vi "VISA test.vi"() -> ()   [LabVIEW 2012]
uses:
  <vilib>/Instr/_visa.llb/VISA Find Search Mode.ctl
  <vilib>/Platform/TimedLoop/XDataNode/timing_clust.ctl
  <vilib>/Platform/TimedLoop/XDataNode/nitl_modes.ctl
  <vilib>/Platform/TimedLoop/XDataNode/wakeup.ctl
  <vilib>/Instr/_visa.llb/VISA Configure Serial Port (Instr).vi
  <vilib>/Platform/TimedLoop/XDataNode/XDataNode.xnode
  <vilib>/Platform/TimedLoop/XDataNode/XDNodeRunTimeDep.lvlib
panel:
  in  "data3":string
  in  "data2":string
  out "Actual polling freq. (Hz)":dbl=10.0
  in  "stop":bool
  in  "Poll freq.(Hz)":dbl=10.0
  in  "data1":string
  in  "cmd":string="2"
  in  "add":u8=1
  out "Checksum ok?":bool=TRUE
  out "chk":u8=183 format="%x"
  out "term":string="\r"
  out "Output to device":string="$012B7\r"
  in  "bytes to read":u32=64
  in  "flow control (0:none)":u16(ring) items=["None", "XON/XOFF", "RTS/CTS", "XON/XOFF & RTS/CTS", "DTR/DSR", "XON/XOFF & DTR/DSR"]
  in  "stop bits":u16(ring)=10 items=["1.0"=10, "1.5"=15, "2.0"=20]
  in  "parity":enum16{"None", "Odd", "Even", "Mark", "Space"}(ring)
  in  "data bits":u16=8 min=5 max=8 step=1
  in  "baud rate (bps)":u32=9600
  in  "timeout (ms)":u32=1000
  in  "enable termination char":bool=TRUE
  in  "termination char":u8=13 format="%.0x"
  out "bytes returned":u32=12
  out "Error":errorcluster
  out "Response from device":string="!010806C0C3\r"
  out "bytes written":u32=7
  in  "del":string="$"
  in  "VISA resource name":refnum<visa-resource-name>="COM3"
  out "Port list":string[](array[string])=["COM1", "COM3"]
  # "(hex)"
  # "(hex)"
  # "(dec)"
  # "(hex)"
  # "(hex)"
  # "(hex)"
  # "(str)"
  # "(str)"
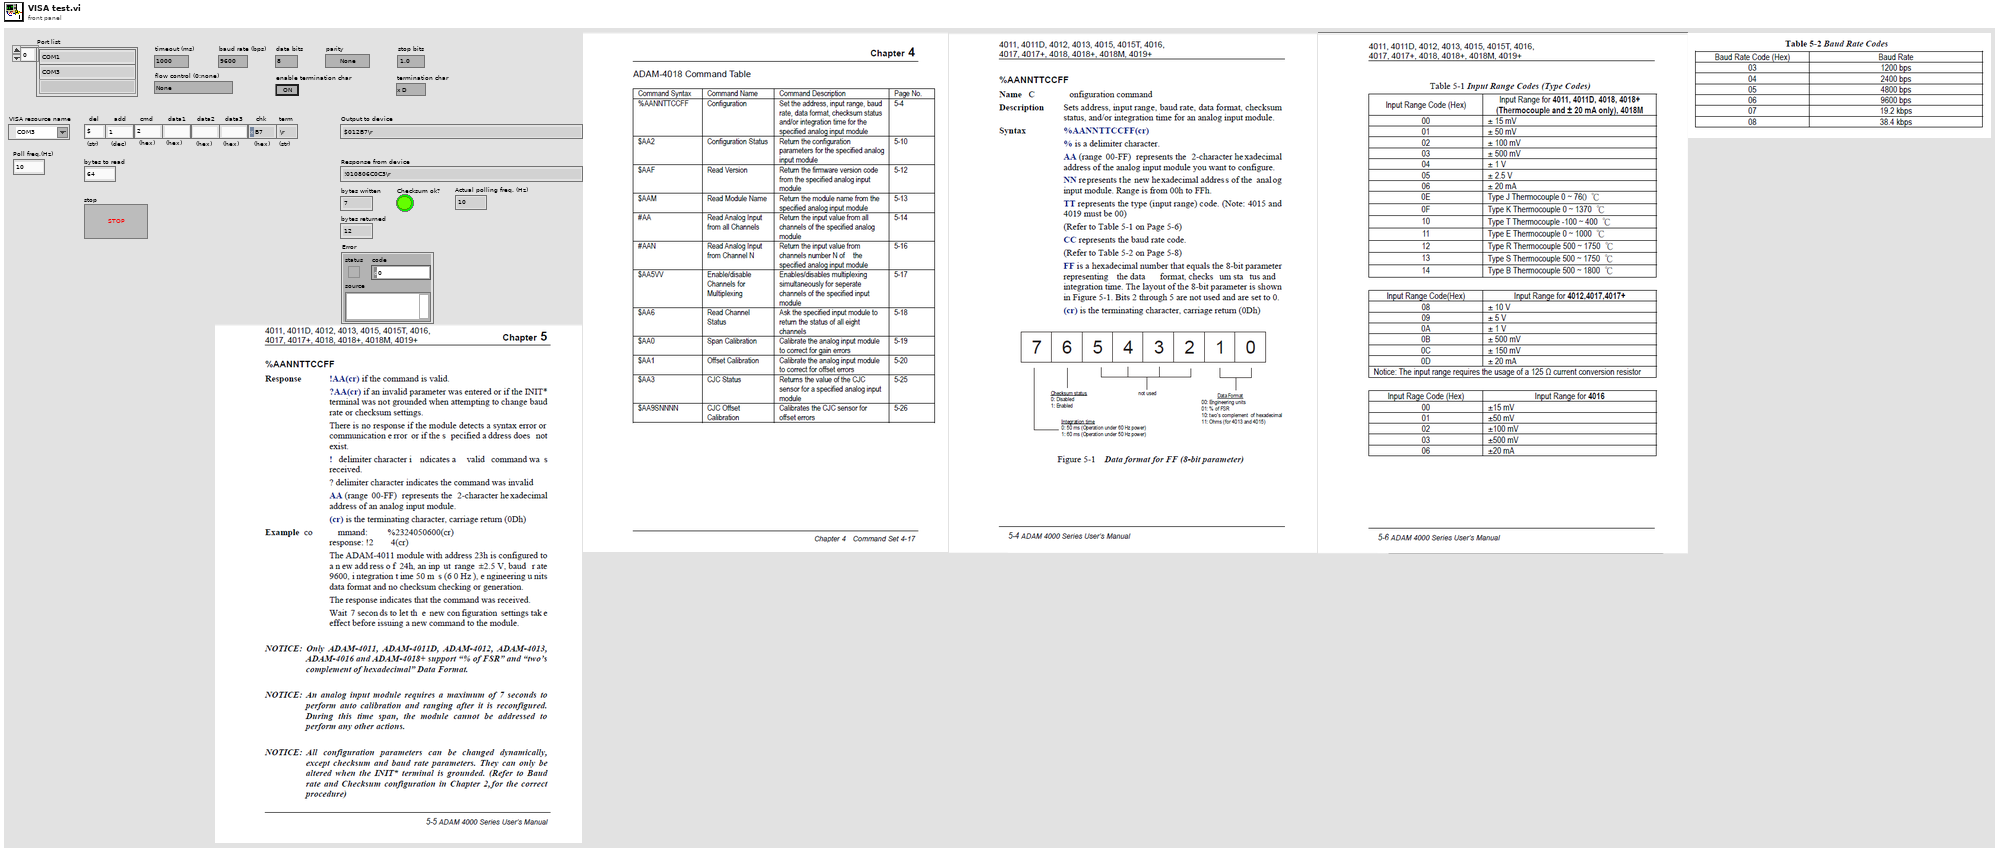
[diagram p1: front panel]
types:
  T1 = typedef "VISA Find Search Mode.ctl" = u32
  T2 = typedef "XDNodeRunTimeDep.lvlib/timing_clust.ctl" = cluster{"Expected End [f-1]":u64, "Actual End [f-1]":u64, "Finished Late? [f-1]":bool, "Expected End [i-1]":u64, "Actual End [i-1]":u64, "Finished Late? [i-1]":bool, "Expected Start [i]":u64, "Actual Start [i]":u64, "Expected Start [f]":u64, "Actual Start [f]":u64, "Source Name":string, "Structure Name":string, "Period":i64, "Deadline":i64, "Offset":i64, "Start":i64, "Priority":i32, "Timeout":i32, "Mode":T3, "Wakeup Reason":T4, "Error":errorcluster, "Source Type":string, "Secondary Source Type":string, "Global End Time":u64, "Global Start Time":u64, "Frame Duration":u64, "Iteration Duration":u64, "Assigned CPU":i32, "I/O Scan Engine Mode":u32}
  T3 = typedef "XDNodeRunTimeDep.lvlib/nitl_modes.ctl" = enum32{"No Change", "Process missed periods, maintain original phase", "Discard missed periods, maintain original phase", "Process missed periods, ignore original phase", "Discard missed periods, ignore original phase"}
  T4 = typedef "XDNodeRunTimeDep.lvlib/wakeup.ctl" = enum32{"Normal", "Aborted", "Asynchronous wakeup", "Timing source error", "Timed loop error", "Timeout"}
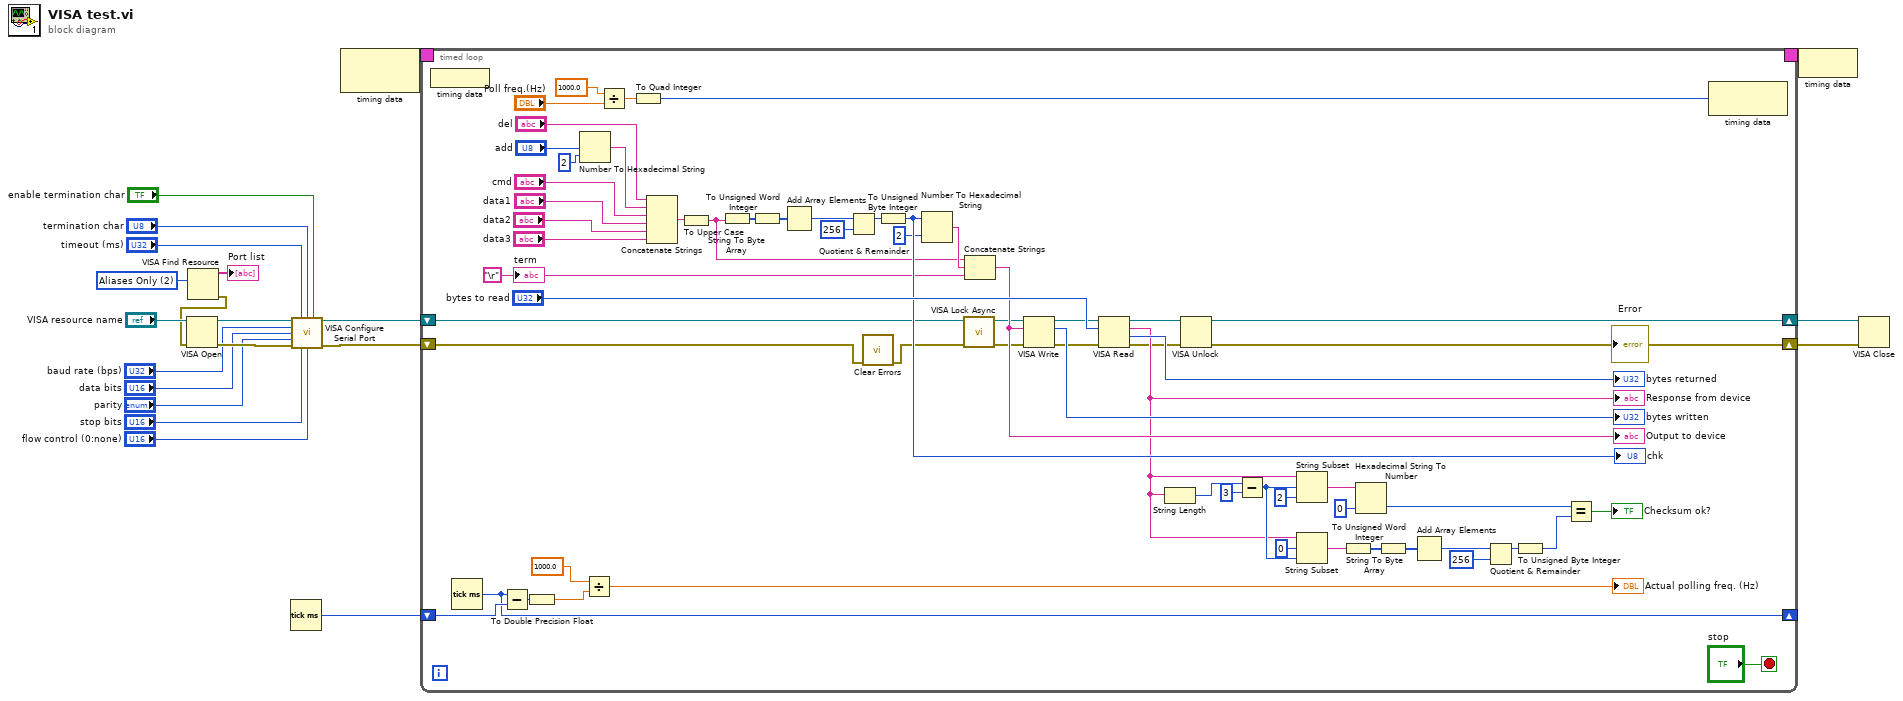
[diagram p0: block diagram]
diagram:
  w20 = T1 2 items=["Canonical Names Only"=0, "Aliases Only"=2, "Include Matching Aliases"=3, "Include All Aliases"=4] ("Search Mode")
  n1 = VISA Find Resource(10:w20) -> (0:w18:errorcluster, 3:→"Port list":string[])  [unwired: 2 in, 1 out]
  n2 = VISA Open(error in (no error)=w18, VISA resource name="VISA resource name") -> (VISA resource name=w17:refnum<visa-resource-name>, error out=w16:errorcluster)  [unwired: 3 in]
  n3 = Tick Count (ms)() -> (millisecond timer value=w1:u32)
  n4 = call-poly "VISA Configure Serial Port"("VISA resource name"=w17, "timeout (10sec)"="timeout (ms)", "termination char\n(0xA = '\\n' = LF)"="termination char", "Enable Termination\nChar (T)"="enable termination char", "baud rate (9600)"="baud rate (bps)", "data bits (8)"="data bits", "parity (0:none)"="parity", "error in (no error)"=w16, "stop bits (10: 1 bit)"="stop bits", "flow control (0:none)"="flow control (0:none)") -> ("VISA resource name out"=w5:refnum<visa-resource-name>, "error out"=w4:errorcluster)  [unwired: 4 in]
  n5 = node-c288() -> (w7:T2)  [unwired: 1 in]
  n6 = timed-loop {
    timing: w7 -> [_]
    timing-out: [_] -> w6
    shift-right: [w43] -> w3
    shift-left: w5 -> [w42]
    shift-right: [w44] -> w2
    shift-left: w4 -> [w23]
    shift-right: [w38] -> _
    shift-left: w1 -> [w39]
    stop <- "stop" stop-if-true
    w65 = "\r"
    n7 = node-c288() -> ()  [unwired: 1 in]
    n8 = Tick Count (ms)() -> (millisecond timer value=w38:u32)
    n9 = Subtract(x=w38, y=w39) -> (x-y=w36:u32)
    n10 = To Double Precision Float(number=w36) -> (double precision float=w35:dbl)
    n11 = Number To Hexadecimal String(1:i16 2 ("width (-)"), 2:"add") -> (0:w58:string)
    n12 = Divide(x=1000.0, y=w35) -> (x/y=→"Actual polling freq. (Hz)":dbl)
    n13 = Divide(x=1000.0, y="Poll freq.(Hz)") -> (x/y=w33:dbl)
    n14 = To Quad Integer(1:w33) -> (0:w30:i64)
    n15 = Concatenate Strings("del", w58, "cmd", "data1", "data2", "data3") -> (w27:string)
    n16 = To Upper Case(1:w27) -> (0:w26:string)
    n17 = String To Byte Array(string=w26) -> (unsigned byte array=w55:u8[])
    n18 = To Unsigned Word Integer(number=w55) -> (unsigned 16bit integer=w54:u16[])
    n19 = Add Array Elements(numeric array=w54) -> (sum=w53:u16)
    n20 = Quotient & Remainder(x=w53, y=u16 256) -> (x-y*floor(x/y)=w62:u16)  [unwired: 1 out]
    n21 = call <vilib>:"Clear Errors.vi"("error in (no error)"=w23) -> ("error out"=w22:errorcluster)  [unwired: 6 in]
    n22 = To Unsigned Byte Integer(number=w62) -> (unsigned 8bit integer=w76:u8)
    "chk" <- w76
    n23 = Number To Hexadecimal String(1:i16 2 ("width (-)"), 2:w76) -> (0:w60:string)
    n24 = call <vilib>:"VISA Lock Async.vi"("error in (no error)"=w22, "VISA resource name"=w42) -> ("error out"=w41:errorcluster, "VISA resource name out"=w40:refnum<visa-resource-name>)  [unwired: 7 in, 1 out]
    n25 = Concatenate Strings(w26, w60, w65) -> (w80:string)
    "Output to device" <- w80
    n26 = VISA Write(VISA resource name=w40, write buffer=w80, error in (no error)=w41) -> (VISA resource name out=w25:refnum<visa-resource-name>, return count=→"bytes written":u32, error out=w24:errorcluster)
    n27 = VISA Read(VISA resource name=w25, byte count="bytes to read", error in (no error)=w24) -> (VISA resource name out=w45:refnum<visa-resource-name>, read buffer=w73:string, return count=→"bytes returned":u32, error out=w46:errorcluster)
    "Response from device" <- w73
    n28 = String Length(string=w73) -> (length=w78:i32)
    n29 = VISA Unlock(8:w46, 11:w45) -> (0:w44:errorcluster, 3:w43:refnum<visa-resource-name>)
    "Error" <- w44
    n30 = Subtract(x=w78, y=3) -> (x-y=w74:i32)
    n31 = String Subset(string=w73, offset (0)=w74, length (rest)=2 ("length (rest)")) -> (substring=w50:string)
    n32 = String Subset(string=w73, offset (0)=0, length (rest)=w74) -> (substring=w72:string)
    n33 = String To Byte Array(string=w72) -> (unsigned byte array=w71:u8[])
    n34 = Hexadecimal String To Number(string=w50, default (0uL)=u8 0 ("default (0 U32)")) -> (number=w48:u8)  [unwired: 1 in, 1 out]
    n35 = To Unsigned Word Integer(number=w71) -> (unsigned 16bit integer=w51:u16[])
    n36 = Add Array Elements(numeric array=w51) -> (sum=w52:u16)
    n37 = Quotient & Remainder(x=w52, y=u16 256) -> (x-y*floor(x/y)=w70:u16)  [unwired: 1 out]
    n38 = To Unsigned Byte Integer(number=w70) -> (unsigned 8bit integer=w68:u8)
    n39 = Equal?(x=w48, y=w68) -> (x = y?=→"Checksum ok?":bool)
    n40 = node-c288(w30) -> ()  [unwired: 1 out]
    "term" <- w65
  }
  n41 = node-c288(w6) -> ()
  n42 = VISA Close(VISA resource name=w3, error in (no error)=w2) -> ()  [unwired: 1 out]
